vi "Main.vi"() -> ()   [LabVIEW 2020, in "String based State machine - Airplane.lvlib"]
doc: "This VI is a Airplane lavatory signs made with the state machine design pattern"
uses:
  String based State machine - Airplane.lvlib
  Typedef/Queue Drive mode.ctl
  Typedef/Data Cluster.ctl
panel:
  out "Error Out":errorcluster
  in  "Stop":bool
  out "Rear Lavatories Occupied":bool caption="Lavatories\nOccupied"
  out "Front Lavatories Occupied":bool caption="Lavatories\nOccupied"
  out "Alarm Timer C":ext caption="secs" format="%#.0f"
  out "Alarm Timer D":ext caption="secs" format="%#.0f"
  out "Lavatory C Return to Seat":bool
  out "Lavatory D Return to Seat":bool
  out "Lavatory C":bool caption="Occupied"
  out "Lavatory D":bool caption="Occupied"
  out "Lavatory B Return to Seat":bool
  out "Lavatory B":bool caption="Occupied"
  out "Alarm Timer B":ext caption="secs" format="%#.0f"
  in  "Alarm Timer Limit":ext caption="secs"
  out "Alarm Timer A":ext caption="secs" format="%#.0f"
  in  "Alarm Acknowledge":bool
  out "Lavatory":string
  out "Alarm":bool
  in  "Seatbelt Sign ON":bool
  out "Lavatory A Return to Seat":bool
  out "Lavatory A":bool caption="Occupied"
  in  "Lavatory D Occupied":bool
  in  "Lavatory C Occupied":bool
  in  "Lavatory B Occupied":bool
  in  "Lavatory A Occupied":bool
  in  "Error In":errorcluster
  # "Airplane Lavatory Signs"
  # "Front"
  # "Rear"
  # "Steward's Area"
  # "Lavatory A"
  # "Lavatory C"
  # "Lavatory B"
  # "Lavatory D"
  # "Simulation Controls & Indicators"
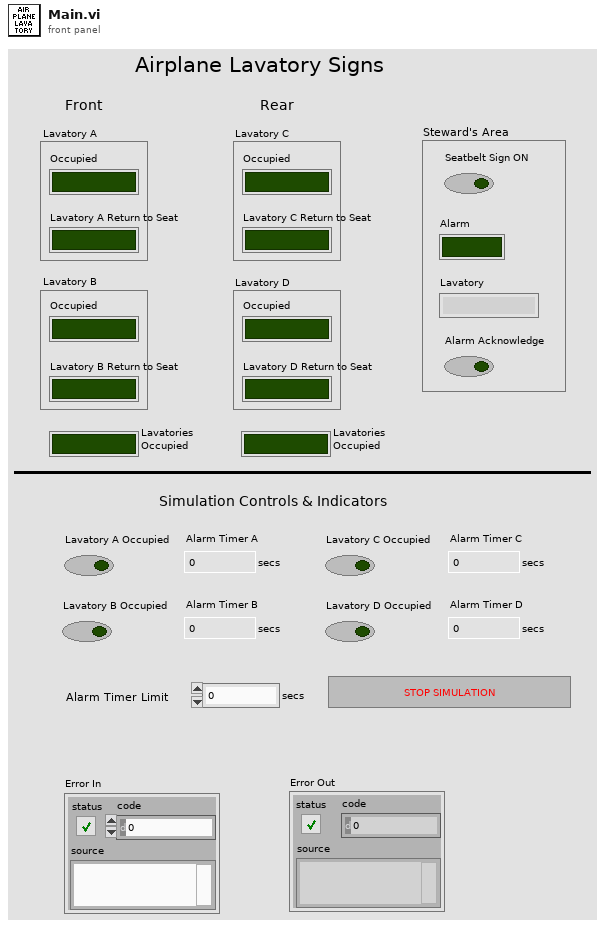
[diagram p1: front panel]
types:
  T1 = typedef "String based State machine - Airplane.lvlib/Data Cluster.ctl" = cluster{"Lavatory A":bool, "Lavatory B":bool, "Lavatory C":bool, "Lavatory D":bool, "Seat belt sign":bool, "Start time A":ext, "A time":ext, "Alarm time alert":ext, "Alarm":bool, "Start":bool, "B time ":ext, "C time ":ext, "D time":ext, "Lavatory":string, "A limit":bool, "B limit":bool, "C limit":bool, "D limit":bool, "Start time B":ext, "Start time C":ext, "Start time D":ext}
  T2 = typedef "String based State machine - Airplane.lvlib/Queue Drive mode.ctl" = enum16{"Create Queue", "Release Queue", "Enqueue N", "Flush Queue", "Enstack", "Dequeue", "Enqueue"}
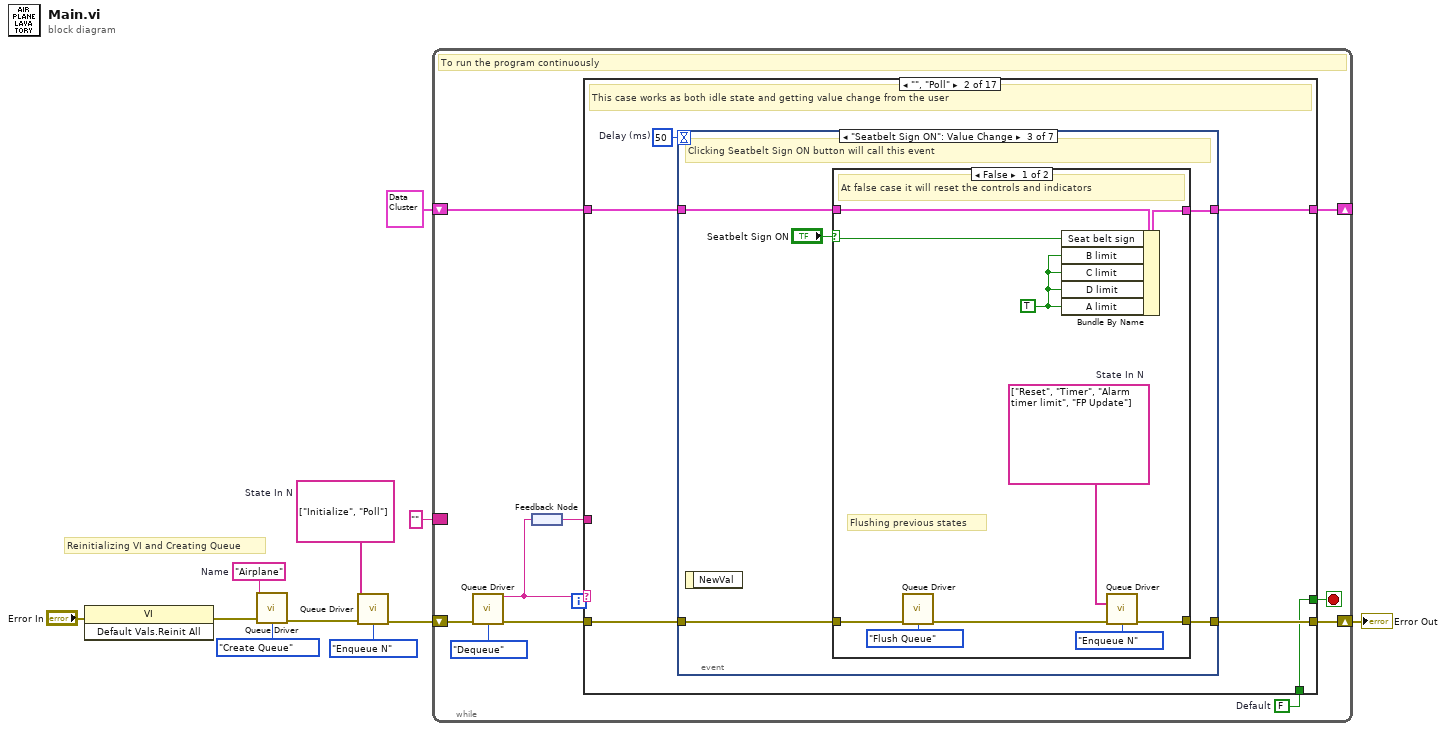
[diagram p0: block diagram]
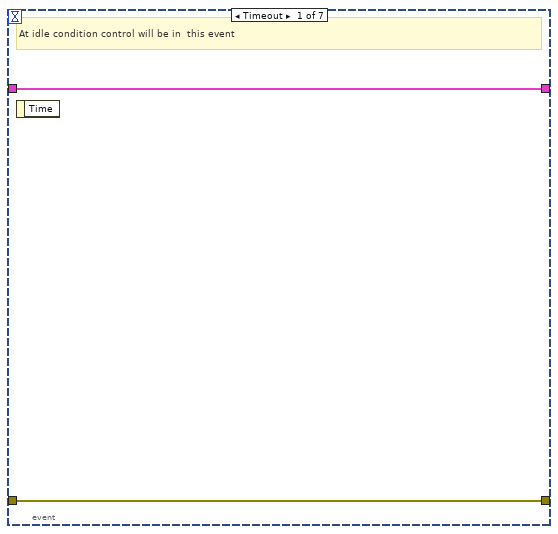
[diagram p3: hidden frame]
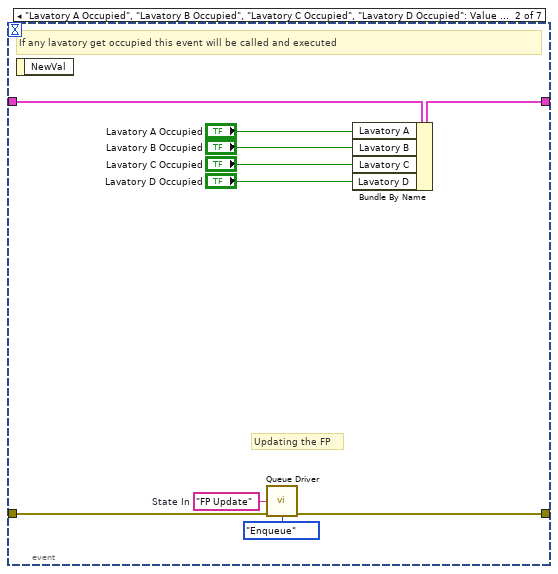
[diagram p4: hidden frame]
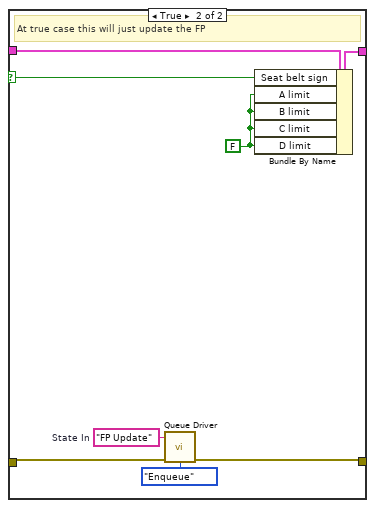
[diagram p5: hidden frame]
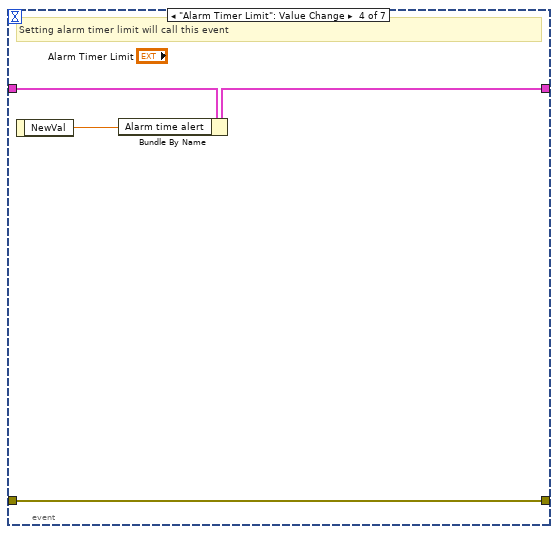
[diagram p6: hidden frame]
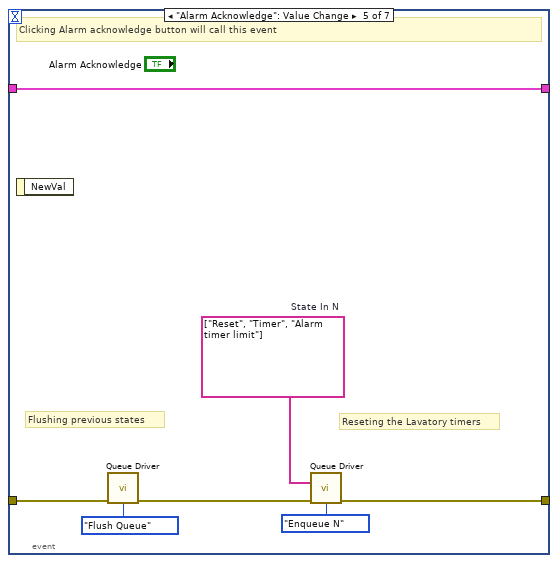
[diagram p7: hidden frame]
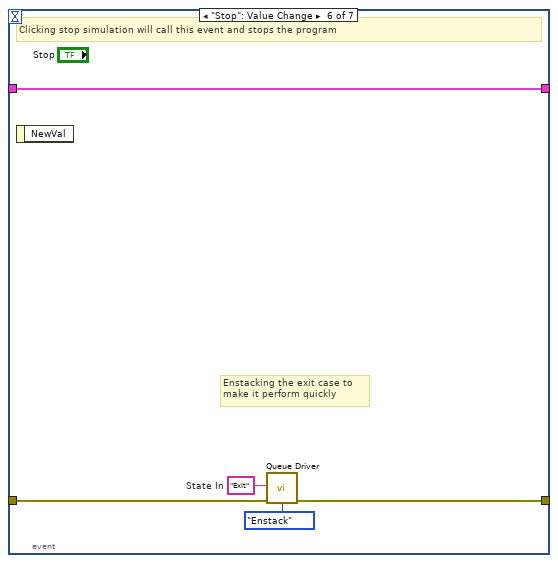
[diagram p8: hidden frame]
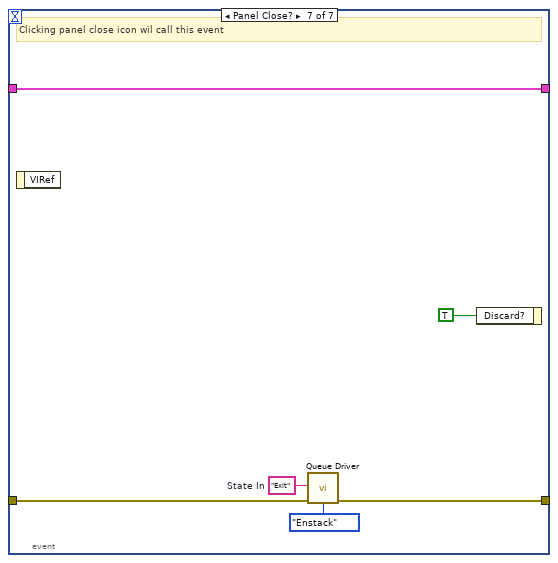
[diagram p9: hidden frame]
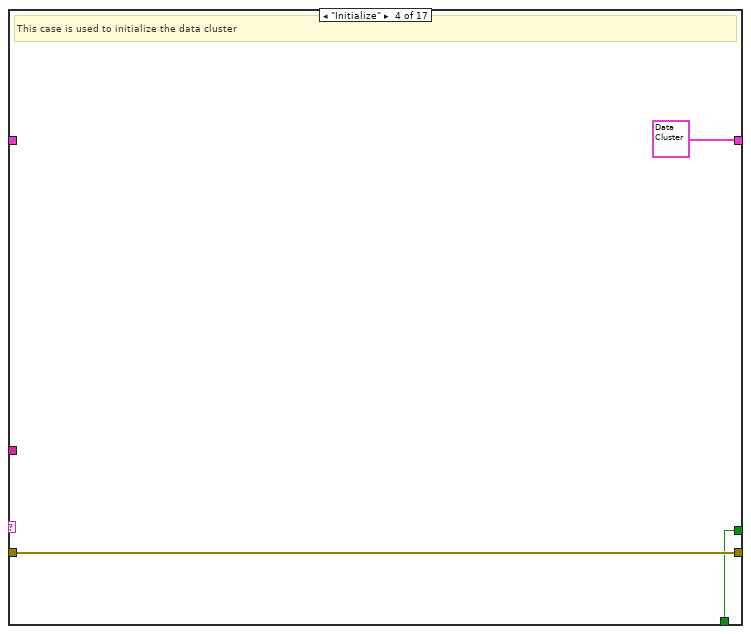
[diagram p11: hidden frame]
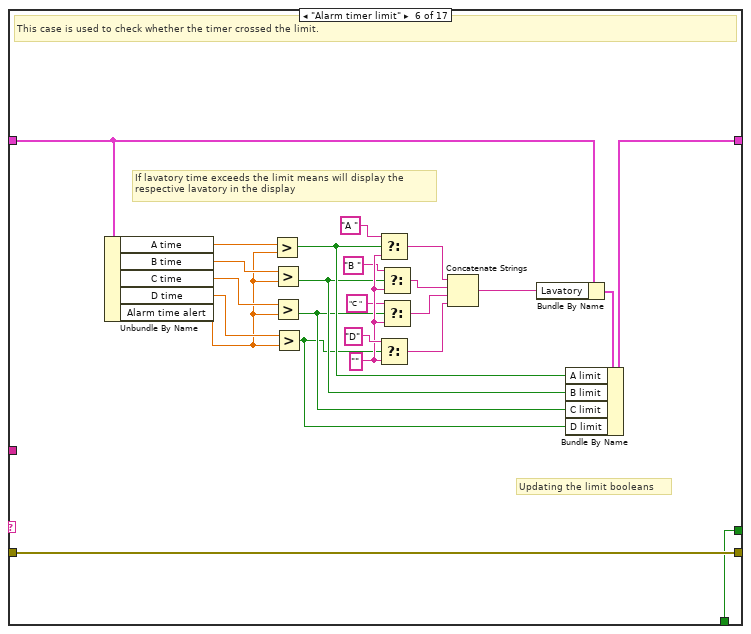
[diagram p13: hidden frame]
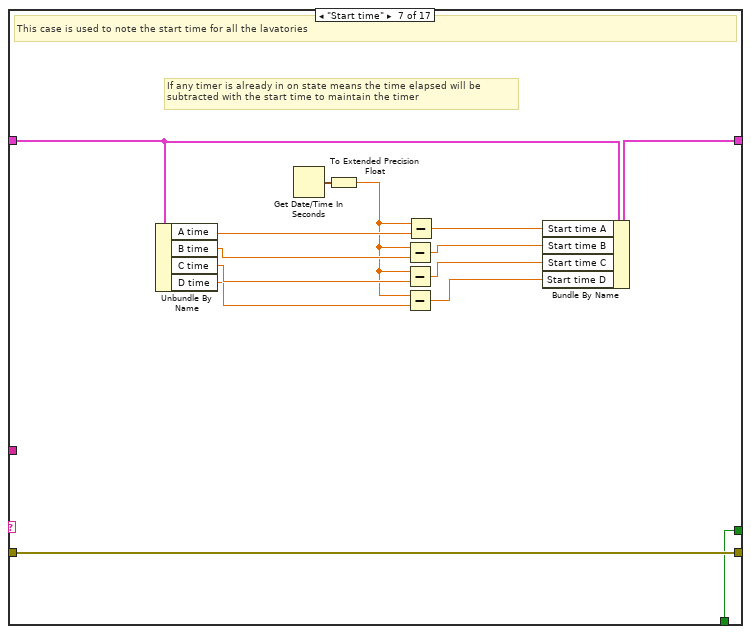
[diagram p14: hidden frame]
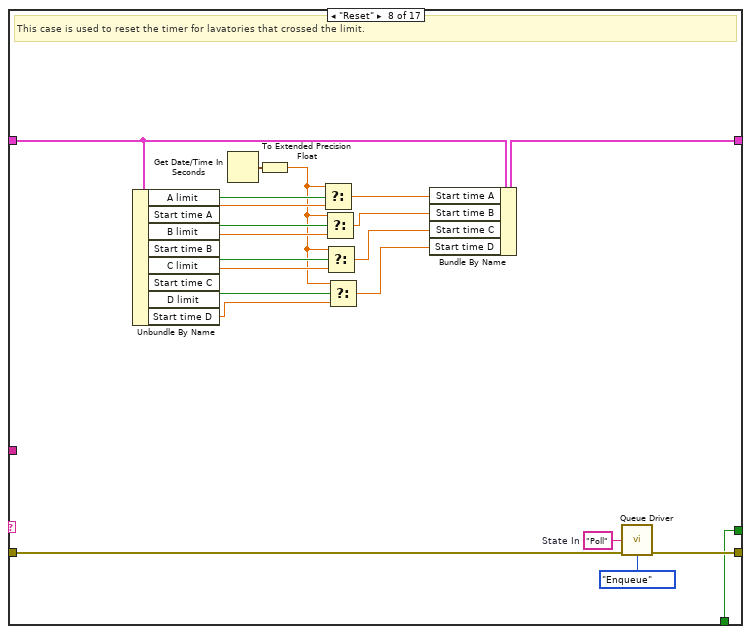
[diagram p15: hidden frame]
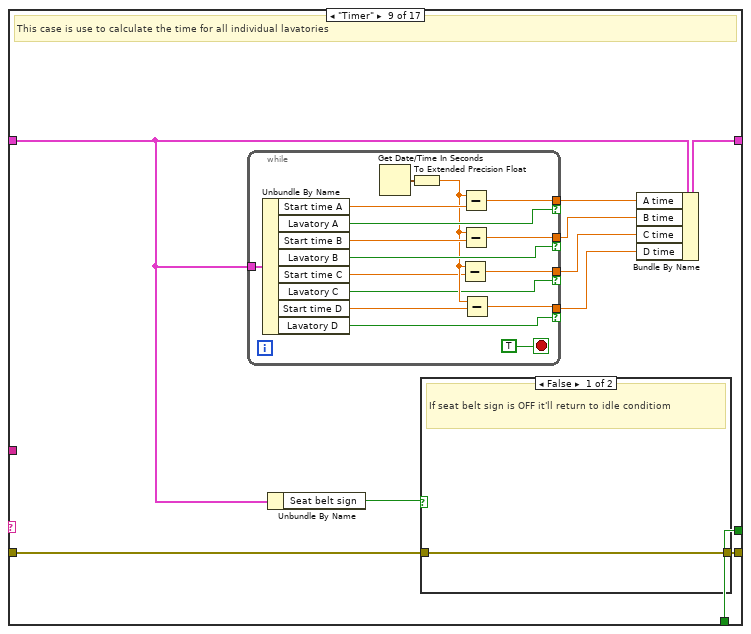
[diagram p16: hidden frame]
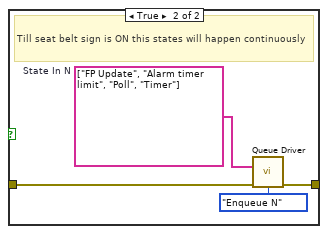
[diagram p17: hidden frame]
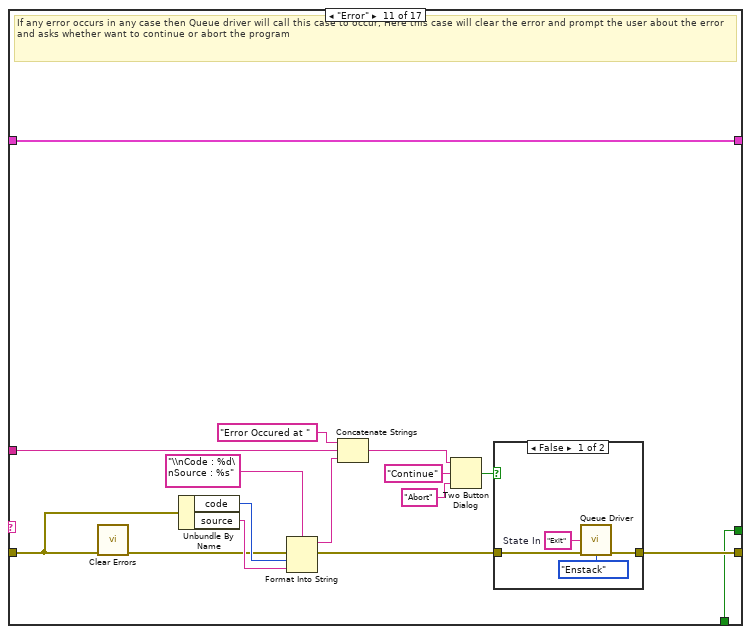
[diagram p19: hidden frame]
diagram:
  w4 = string[] ["Initialize", "Poll"]  # State In N
  w9 = "Airplane"  # Name
  # "Reinitializing VI and Creating Queue"
  n1 = invoke class="VI" method="Default Vals.Reinit All"(error in="Error In") -> (error out=w7:errorcluster)  [unwired: 2 in, 2 out]
  n2 = call "Queue Driver.vi"("Name"=w9, "Error In"=w7, "Enum"=Queue_Drive_mode."Create Queue") -> ("Error Out"=w11:errorcluster)  [unwired: 11 in, 1 out]
  n3 = call "Queue Driver.vi"("State In N"=w4, "Error In"=w11, "Enum"=Queue_Drive_mode."Enqueue N") -> ("Error Out"=w10:errorcluster)  [unwired: 11 in, 1 out]
  n4 = while {
    shift-right: [w18] -> _
    shift-left: T1 {"Lavatory A"=FALSE, "Lavatory B"=FALSE, "Lavatory C"=FALSE, "Lavatory D"=FALSE, "Seat belt sign"=FALSE, "Start time A"=0.0, "A time"=0.0, "Alarm time alert"=0.0, "Alarm"=FALSE, "Start"=FALSE, "B time "=0.0, "C time "=0.0, "D time"=0.0, "Lavatory"="", "A limit"=FALSE, "B limit"=FALSE, "C limit"=FALSE, "D limit"=FALSE, "Start time B"=0.0, "Start time C"=0.0, "Start time D"=0.0} ("Data Cluster") -> [w19]
    shift-right: [w20] -> w5
    shift-left: w10 -> [w21]
    border: "" ("State Out") -> [_]
    stop <- w17 stop-if-true
    w13 = FALSE  # Default
    # "To run the program continuously"
    n5 = call "Queue Driver.vi"("Error In"=w21, "Enum"=Queue_Drive_mode."Dequeue") -> ("State Out"=w16:string, "Error Out"=w15:errorcluster)  [unwired: 12 in]
    n6 = feedback-in #1(w16) -> ()
    n7 = feedback #1() -> (w14:string)
    n8 = case shown="\"\", \"Poll\"" w16 {
      selector: w16 -> [_ _ _ _ _ _ _ _ _ _ _ _ w215 _ _ _ _]
      tunnel: w15 -> [w24 w29 w90 w93 w96 w120 w123 w140 w161 w189 w190 w213 w216 w220 w232 w250 w255]
      tunnel: [w24 w30 w90 w93 w96 w120 w123 w141 w163 w189 w198 w213 w216 w220 w241 w250 w253] -> w20
      tunnel: w19 -> [w23 w27 w89 _ w95 w106 w132 w146 w157 w188 w205 w212 w217 w219 w242 w249 w257]
      tunnel: [w23 w28 w89 T1 {"Lavatory A"=FALSE, "Lavatory B"=FALSE, "Lavatory C"=FALSE, "Lavatory D"=FALSE, "Seat belt sign"=FALSE, "Start time A"=0.0, "A time"=0.0, "Alarm time alert"=0.0, "Alarm"=FALSE, "Start"=FALSE, "B time "=0.0, "C time "=0.0, "D time"=0.0, "Lavatory"=" ", "A limit"=FALSE, "B limit"=FALSE, "C limit"=FALSE, "D limit"=FALSE, "Start time B"=0.0, "Start time C"=0.0, "Start time D"=0.0} ("Data Cluster") w95 w104 w131 w147 w165 w188 w205 w212 w217 w219 w242 w249 w257] -> w18
      tunnel: [w22 w25 w88 w91 w94 w97 w121 w136 w156 w187 w197 w211 w214 w218 w221 w248 TRUE] -> w17
      tunnel: w14 -> [_ _ _ _ _ _ _ _ _ _ w201 _ _ _ _ _ _]
      tunnel: w13 -> [w22 w25 w88 w91 w94 w97 w121 w136 w156 w187 w197 w211 _ w218 w221 w248 _]
      frame "/*****Poll*****/" {
      }
      frame "", "Poll" {
        w26 = 50  # Delay (ms)
        # "This case works as both idle state and getting value change from the user"
        n9 = event shown="[2] \"Seatbelt Sign ON\": Value Change" {
          selector: _ -> [_ _ _ _ _ _ _]
          dyn-events: _ -> [_ _ _ _ _ _ _]
          timeout: w26 -> [_ _ _ _ _ _ _]
          tunnel: [w31 w36 w47 w66 w75 w80 w85] -> w30
          tunnel: w29 -> [w31 w35 w46 w66 w73 w79 w84]
          tunnel: [w32 w42 w43 w69 w76 w81 w87] -> w28
          tunnel: w27 -> [w32 w37 w45 w68 w76 w81 w87]
          event Timeout {
            # "At idle condition control will be in  this event"
            n10 = event-data() -> ()  [unwired: 1 in, 1 out]
          }
          event "Lavatory A Occupied", "Lavatory B Occupied", "Lavatory C Occupied", "Lavatory D Occupied": Value Change {
            w34 = "FP Update"  # State In
            # "Updating the FP"
            # "If any lavatory get occupied this event will be called and executed"
            n11 = event-data() -> ()  [unwired: 1 in, 1 out]
            n12 = call "Queue Driver.vi"("State In"=w34, "Error In"=w35, "Enum"=Queue_Drive_mode."Enqueue") -> ("Error Out"=w36:errorcluster)  [unwired: 11 in, 1 out]
            n13 = Bundle By Name(cluster=w37, "Lavatory A"="Lavatory A Occupied", "Lavatory B"="Lavatory B Occupied", "Lavatory C"="Lavatory C Occupied", "Lavatory D"="Lavatory D Occupied") -> (w42:T1)
          }
          event "Seatbelt Sign ON": Value Change {
            # "Clicking Seatbelt Sign ON button will call this event"
            n14 = event-data() -> ()  [unwired: 1 in, 1 out]
            n15 = case shown="False" "Seatbelt Sign ON" {
              selector: "Seatbelt Sign ON" -> [w52 w61]
              tunnel: [w57 w65] -> w47
              tunnel: w46 -> [w50 w64]
              tunnel: w45 -> [w55 w63]
              tunnel: [w54 w62] -> w43
              frame False {
                w53 = TRUE ("A limit")
                w56 = string[] ["Reset", "Timer", "Alarm timer limit", "FP Update"]  # State In N
                # "Flushing previous states"
                # "At false case it will reset the controls and indicators"
                n16 = call "Queue Driver.vi"("Error In"=w50, "Enum"=Queue_Drive_mode."Flush Queue") -> ("Error Out"=w51:errorcluster)  [unwired: 12 in, 1 out]
                n17 = Bundle By Name(cluster=w55, "Seat belt sign"=w52, "B limit"=w53, "C limit"=w53, "D limit"=w53, "A limit"=w53) -> (w54:T1)
                n18 = call "Queue Driver.vi"("State In N"=w56, "Error In"=w51, "Enum"=Queue_Drive_mode."Enqueue N") -> ("Error Out"=w57:errorcluster)  [unwired: 11 in, 1 out]
              }
              frame True {
                w59 = FALSE ("A limit")
                w60 = "FP Update"  # State In
                # "At true case this will just update the FP"
                n19 = call "Queue Driver.vi"("State In"=w60, "Error In"=w64, "Enum"=Queue_Drive_mode."Enqueue") -> ("Error Out"=w65:errorcluster)  [unwired: 11 in, 1 out]
                n20 = Bundle By Name(cluster=w63, "Seat belt sign"=w61, "A limit"=w59, "B limit"=w59, "C limit"=w59, "D limit"=w59) -> (w62:T1)
              }
            }
          }
          event "Alarm Timer Limit": Value Change {
            # "Setting alarm timer limit will call this event"
            n21 = event-data() -> ("NewVal"=w67:ext)  [unwired: 1 in]
            n22 = Bundle By Name(cluster=w68, "Alarm time alert"=w67) -> (w69:T1)
          }
          event "Alarm Acknowledge": Value Change {
            w72 = string[] ["Reset", "Timer", "Alarm timer limit"]  # State In N
            # "Reseting the Lavatory timers"
            # "Flushing previous states"
            # "Clicking Alarm acknowledge button will call this event"
            n23 = event-data() -> ()  [unwired: 1 in, 1 out]
            n24 = call "Queue Driver.vi"("Error In"=w73, "Enum"=Queue_Drive_mode."Flush Queue") -> ("Error Out"=w74:errorcluster)  [unwired: 12 in, 1 out]
            n25 = call "Queue Driver.vi"("State In N"=w72, "Error In"=w74, "Enum"=Queue_Drive_mode."Enqueue N") -> ("Error Out"=w75:errorcluster)  [unwired: 11 in, 1 out]
          }
          event "Stop": Value Change {
            w78 = "Exit"  # State In
            # "Enstacking the exit case to\nmake it perform quickly"
            # "Clicking stop simulation will call this event and stops the program"
            n26 = event-data() -> ()  [unwired: 1 in, 1 out]
            n27 = call "Queue Driver.vi"("State In"=w78, "Error In"=w79, "Enum"=Queue_Drive_mode."Enstack") -> ("Error Out"=w80:errorcluster)  [unwired: 11 in, 1 out]
          }
          event Panel Close? {
            w83 = "Exit"  # State In
            # "Clicking panel close icon wil call this event"
            n28 = event-data() -> ()  [unwired: 1 in, 1 out]
            n29 = call "Queue Driver.vi"("State In"=w83, "Error In"=w84, "Enum"=Queue_Drive_mode."Enstack") -> ("Error Out"=w85:errorcluster)  [unwired: 11 in, 1 out]
            n30 = event-data("Discard?"=TRUE) -> ()  [unwired: 1 in, 1 out]
          }
        }
      }
      frame "/*****Initialize*****/" {
      }
      frame "Initialize" {
        # "This case is used to initialize the data cluster"
      }
      frame "/*****Timer*****/" {
      }
      frame "Alarm timer limit" {
        w112 = "" ("f")
        # "If lavatory time exceeds the limit means will display the \nrespective lavatory in the display"
        # "Updating the limit booleans"
        # "This case is used to check whether the timer crossed the limit."
        n31 = Unbundle By Name(w106) -> ("A time"=w119:ext, "B time"=w118:ext, "C time"=w117:ext, "D time"=w116:ext, "Alarm time alert"=w115:ext)
        n32 = Greater?(x=w119, y=w115) -> (0:w103:bool)
        n33 = Greater?(x=w118, y=w115) -> (0:w102:bool)
        n34 = Greater?(x=w117, y=w115) -> (0:w101:bool)
        n35 = Greater?(x=w116, y=w115) -> (0:w100:bool)
        n36 = Select(t="A " ("State In"), s=w103, f=w112) -> (s? t:f=w110:string)
        n37 = Select(t="D" ("State In"), s=w100, f=w112) -> (s? t:f=w107:string)
        n38 = Select(t="B " ("State In"), s=w102, f=w112) -> (s? t:f=w109:string)
        n39 = Select(t="C ", s=w101, f=w112) -> (s? t:f=w108:string)
        n40 = Concatenate Strings(w110, w109, w108, w107) -> (w99:string)
        n41 = Bundle By Name(cluster=w106, "Lavatory"=w99) -> (w105:T1)
        n42 = Bundle By Name(cluster=w105, "A limit"=w103, "B limit"=w102, "C limit"=w101, "D limit"=w100) -> (w104:T1)
      }
      frame "Start time" {
        # "If any timer is already in on state means the time elapsed will be\nsubtracted with the start time to maintain the timer"
        # "This case is used to note the start time for all the lavatories"
        n43 = Unbundle By Name(w132) -> ("A time"=w134:ext, "B time"=w133:ext, "C time"=w127:ext, "D time"=w126:ext)
        n44 = Get Date/Time In Seconds() -> (seconds since 1Jan1904=w128:timestamp)
        n45 = To Extended Precision Float(1:w128) -> (0:w122:ext)
        n46 = Subtract(x=w122, y=w133) -> (x-y=w129:ext)
        n47 = Subtract(x=w122, y=w127) -> (x-y=w125:ext)
        n48 = Subtract(x=w122, y=w126) -> (x-y=w124:ext)
        n49 = Subtract(x=w122, y=w134) -> (x-y=w130:ext)
        n50 = Bundle By Name(cluster=w132, "Start time A"=w130, "Start time B"=w129, "Start time C"=w125, "Start time D"=w124) -> (w131:T1)
      }
      frame "Reset" {
        w139 = "Poll"  # State In
        # "This case is used to reset the timer for lavatories that crossed the limit."
        n51 = Unbundle By Name(w146) -> ("A limit"=w155:bool, "Start time A"=w154:ext, "B limit"=w153:bool, "Start time B"=w152:ext, "C limit"=w151:bool, "Start time C"=w150:ext, "D limit"=w149:bool, "Start time D"=w148:ext)
        n52 = Get Date/Time In Seconds() -> (seconds since 1Jan1904=w138:timestamp)
        n53 = To Extended Precision Float(1:w138) -> (0:w137:ext)
        n54 = Select(t=w137, s=w155, f=w154) -> (s? t:f=w145:ext)
        n55 = Select(t=w137, s=w153, f=w152) -> (s? t:f=w144:ext)
        n56 = Select(t=w137, s=w151, f=w150) -> (s? t:f=w143:ext)
        n57 = Select(t=w137, s=w149, f=w148) -> (s? t:f=w142:ext)
        n58 = Bundle By Name(cluster=w146, "Start time A"=w145, "Start time B"=w144, "Start time C"=w143, "Start time D"=w142) -> (w147:T1)
        n59 = call "Queue Driver.vi"("State In"=w139, "Error In"=w140, "Enum"=Queue_Drive_mode."Enqueue") -> ("Error Out"=w141:errorcluster)  [unwired: 11 in, 1 out]
      }
      frame "Timer" {
        # "This case is use to calculate the time for all individual lavatories"
        n60 = while {
          tunnel: w157 -> [w181]
          tunnel: [w178] -> w164 if=w177
          tunnel: [w175] -> w162 if=w174
          tunnel: [w169] -> w160 if=w167
          tunnel: [w168] -> w159 if=w166
          stop <- TRUE stop-if-true
          n61 = Unbundle By Name(w181) -> ("Start time A"=w179:ext, "Lavatory A"=w177:bool, "Start time B"=w176:ext, "Lavatory B"=w174:bool, "Start time C"=w171:ext, "Lavatory C"=w167:bool, "Start time D"=w170:ext, "Lavatory D"=w166:bool)
          n62 = Get Date/Time In Seconds() -> (seconds since 1Jan1904=w180:timestamp)
          n63 = To Extended Precision Float(1:w180) -> (0:w172:ext)
          n64 = Subtract(x=w172, y=w171) -> (x-y=w169:ext)
          n65 = Subtract(x=w172, y=w179) -> (x-y=w178:ext)
          n66 = Subtract(x=w172, y=w176) -> (x-y=w175:ext)
          n67 = Subtract(x=w172, y=w170) -> (x-y=w168:ext)
        }
        n68 = Unbundle By Name(w157) -> ("Seat belt sign"=w158:bool)
        n69 = case shown="False" w158 {
          tunnel: [w182 w186] -> w163
          tunnel: w161 -> [w182 w185]
          frame False {
            # "If seat belt sign is OFF it'll return to idle conditiom"
          }
          frame True {
            w184 = string[] ["FP Update", "Alarm timer limit", "Poll", "Timer"]  # State In N
            # "Till seat belt sign is ON this states will happen continuously"
            n70 = call "Queue Driver.vi"("State In N"=w184, "Error In"=w185, "Enum"=Queue_Drive_mode."Enqueue N") -> ("Error Out"=w186:errorcluster)  [unwired: 11 in, 1 out]
          }
        }
        n71 = Bundle By Name(cluster=w157, "A time"=w164, "B time"=w162, "C time"=w160, "D time"=w159) -> (w165:T1)
      }
      frame "/*****Error*****/" {
      }
      frame "Error" {
        # "If any error occurs in any case then Queue driver will call this case to occur, Here this case will clear the error and prompt the user about the error and asks whether want to continue or abort the program"
        n72 = call <vilib>:"Clear Errors.vi"("error in (no error)"=w190) -> ("error out"=w191:errorcluster)  [unwired: 5 in, 1 out]
        n73 = Unbundle By Name(w190) -> ("code"=w194:i32, "source"=w195:string)
        n74 = Format Into String(format string="\\nCode : %d\nSource : %s", error in=w191, w194, w195) -> (resulting string=w192:string, error out=w196:errorcluster)  [unwired: 1 in]
        n75 = Concatenate Strings("Error Occured at " ("string"), w201, w192) -> (w200:string)
        n76 = Two Button Dialog(message=w200, 1:"Abort" ("F button name (\"Cancel\")"), 2:"Continue" ("T button name (\"OK\")")) -> (T button?=w199:bool)
        n77 = case shown="False" w199 {
          tunnel: [w209 w210] -> w198
          tunnel: w196 -> [w208 w210]
          frame False {
            w207 = "Exit"  # State In
            n78 = call "Queue Driver.vi"("State In"=w207, "Error In"=w208, "Enum"=Queue_Drive_mode."Enstack") -> ("Error Out"=w209:errorcluster)  [unwired: 11 in, 1 out]
          }
          frame True {
          }
        }
      }
      frame "/*****Default*****/" {
      }
      frame Default {
        # "Any other case names will be execute this event and prompt the user."
        n79 = One Button Dialog(message=w215) -> (true=w214:bool)  [unwired: 1 in]
      }
      frame "/*****Front Panel*****/" {
      }
      frame "FP Update" {
        # "Calls timer when seat belt is ON or it'll \ngo to idle state."
        # "This case is used to update the indicators in the FP."
        n80 = Unbundle By Name(w242) -> ("A limit"=w233:bool, "B limit"=w234:bool, "C limit"=w235:bool, "D limit"=w236:bool, "Seat belt sign"=w222:bool, "Lavatory A"=w228:bool, "Lavatory B"=w227:bool, "Lavatory C"=w225:bool, "Lavatory D"=w224:bool, "A time"=→"Alarm Timer A":ext, "B time"=→"Alarm Timer B":ext, "C time"=→"Alarm Timer C":ext, "D time"=→"Alarm Timer D":ext, "Lavatory"=→"Lavatory":string)
        "Lavatory A Return to Seat" <- w222
        "Lavatory A" <- w228
        "Lavatory B" <- w227
        "Lavatory B Return to Seat" <- w222
        "Lavatory C" <- w225
        "Lavatory D" <- w224
        "Lavatory C Return to Seat" <- w222
        "Lavatory D Return to Seat" <- w222
        n81 = Compound Arithmetic op=OR(w233, w234, w235, w236) -> (w231:bool)
        n82 = case shown="True" w222 {
          tunnel: [w243 w247] -> w241
          tunnel: w232 -> [w243 w246]
          frame False {
          }
          frame True {
            w245 = string[] ["Start time", "Timer"]  # State In N
            n83 = call "Queue Driver.vi"("State In N"=w245, "Error In"=w246, "Enum"=Queue_Drive_mode."Enqueue N") -> ("Error Out"=w247:errorcluster)  [unwired: 11 in, 1 out]
          }
        }
        n84 = And(x=w231, y=w222) -> (x .and. y?=→"Alarm":bool)
        n85 = And(x=w228, y=w227) -> (x .and. y?=→"Front Lavatories Occupied":bool)
        n86 = And(x=w225, y=w224) -> (x .and. y?=→"Rear Lavatories Occupied":bool)
      }
      frame "/*****Exit*****/" {
      }
      frame "Exit" {
        # "Flushing the previous states and releasing the queue"
        # "Used to terminate the program"
        n87 = call "Queue Driver.vi"("Error In"=w255, "Enum"=Queue_Drive_mode."Flush Queue") -> ("Error Out"=w254:errorcluster)  [unwired: 12 in, 1 out]
        n88 = call "Queue Driver.vi"("Error In"=w254, "Enum"=Queue_Drive_mode."Release Queue") -> ("Error Out"=w253:errorcluster)  [unwired: 12 in, 1 out]
      }
    }
  }
  "Error Out" <- w5
